vi "PH_Beamline_Chief.switch Exp Shutters.vi"(0 "i ref in":refnum<vi>, 1 "Status Subscriber Information before":T1, 5 "error in":errorcluster) -> (14 "i ref out":refnum<vi>, 19 "error out":errorcluster)   [LabVIEW 2014, in "PH_Beamline_Chief.lvlib"]
doc: "This VI sets the Switch GUI State GUI object."
uses:
  PH_Beamline_Chief.lvlib
  PH_Beamline/PH_Beamline.Status Subscriber Information.ctl
  PH_BL-Master/PH_BL-Master.Status Subscriber Information.ctl
  PH_BL-Master/PH_BL-Master.Attribute Set.ctl
  PH_Beamline/PH_Beamline.Switch Instances.ctl
  PH_Beamline/PH_Beamline.lvlib
  PH_Classes/PH_Switch/PH_Switch.lvlib
  PH_BL-Master/PH_BL-Master.lvlib
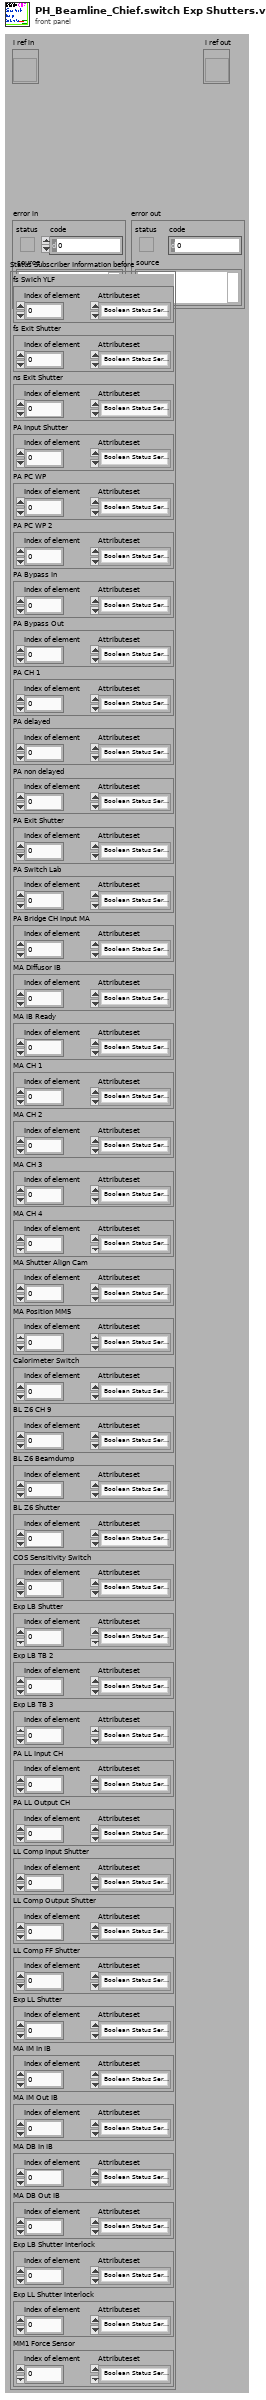
[diagram p1: front panel]
types:
  T1 = typedef "PH_Beamline.lvlib/PH_Beamline.Status Subscriber Information.ctl" = cluster{"fs Swich YLF":T2, "fs Exit Shutter":T2, "ns Exit Shutter":T2, "PA Input Shutter":T2, "PA PC WP":T2, "PA PC WP 2":T2, "PA Bypass In":T2, "PA Bypass Out":T2, "PA CH 1":T2, "PA delayed":T2, "PA non delayed":T2, "PA Exit Shutter":T2, "PA Switch Lab":T2, "PA Bridge CH Input MA":T2, "MA Diffusor IB":T2, "MA IB Ready":T2, "MA CH 1":T2, "MA CH 2":T2, "MA CH 3":T2, "MA CH 4":T2, "MA Shutter Align Cam":T2, "MA Position MM5":T2, "Calorimeter Switch":T2, "BL Z6 CH 9":T2, "BL Z6 Beamdump":T2, "BL Z6 Shutter":T2, "COS Sensitivity Switch":T2, "Exp LB Shutter":T2, "Exp LB TB 2":T2, "Exp LB TB 3":T2, "PA LL Input CH":T2, "PA LL Output CH":T2, "LL Comp Input Shutter":T2, "LL Comp Output Shutter":T2, "LL Comp FF Shutter":T2, "Exp LL Shutter":T2, "MA IM In IB":T2, "MA IM Out IB":T2, "MA DB In IB":T2, "MA DB Out IB":T2, "Exp LB Shutter Interlock":T2, "Exp LL Shutter Interlock":T2, "MM1 Force Sensor":T2}
  T2 = typedef "PH_BL-Master.lvlib/PH_BL-Master.Status Subscriber Information.ctl" = cluster{"Index of element":i32, "Attributeset":T3}
  T3 = typedef "PH_BL-Master.lvlib/PH_BL-Master.Attribute Set.ctl" = enum16{"Boolean Status Service Subscriber", "Picture Status Service Subscriber"}
  T4 = typedef "PH_Beamline.lvlib/PH_Beamline.Switch Instances.ctl" = string
  T5 = typedef "PH_Beamline.lvlib/PH_Beamline.i attribute.ctl" = cluster{"GUI Refs":cluster{"PA ok":refnum<vi>, "MA ok":refnum<vi>, "fs FE ok":refnum<vi>, "ns FE ok":refnum<vi>, "PA ED ok":refnum<vi>, "MAS ok":refnum<vi>, "Booster ok":refnum<vi>, "Mirrortower ok":refnum<vi>, "In.-Box ok":refnum<vi>, "Compressor ok":refnum<vi>, "Experiment LB ok":refnum<vi>, "Experiment LL ok":refnum<vi>, "PHELIX_Beckhoff_Watchdog":refnum<vi>, "Shutters closed":refnum<vi>, "uOPA ok":refnum<vi>, "Vacuum no shotcond Comp LB":refnum<vi>}, "Refs BL MA":refnum<vi>[], "Refs BL MA-IB":refnum<vi>[], "Refs BL fs":refnum<vi>[], "Refs BL PA ED":refnum<vi>[], "Refs BL MAS":refnum<vi>[], "Refs BL Boo":refnum<vi>[], "Refs BL ns":refnum<vi>[], "Refs BL Mirrortower":refnum<vi>[], "Refs BL Compressor":refnum<vi>[], "Refs BL Exp LB":refnum<vi>[], "Radiation Safety":cluster{"Exp Laserbay":cluster{"Ref Op Mode":refnum<vi>, "Ref Laserbay evacuated":refnum<vi>, "Tagname LB evacuated":string, "Shot Mode":T6, "Laserbay evacuated?":i32, "Tagname HV room locked":string, "HV room locked?":i32, "Ref HV room locked":refnum<vi>, "Tagname bridged?":string, "Ref Bridge":refnum<vi>, "I<1E18W/cm²":bool}, "Exp Laserlab":cluster{"Ref Op Mode":refnum<vi>, "Ref Laserlab evacuated":refnum<vi>, "Tagname LL evacuated":string, "Shot Mode":T6, "Laserlab evacuated?":i32, "Tagname bridged?":string, "Ref Bridge":refnum<vi>, "I<1E18W/cm²":bool}}, "Refs BL LL":refnum<vi>[], "PP Igni Heating GUI Refs":refnum<vi>[], "PP Igni Heating Tagnames ":string[], "Refs BL PA":cluster{"undelayed Line before Shutter":refnum<vi>[], "undelayed Line after Shutter":refnum<vi>[], "before Bypass":refnum<vi>[], "delayed Line before Shutter":refnum<vi>[], "delayed Line after Shutter":refnum<vi>[], "before Shutter Input":refnum<vi>[], "after Shutter Input":refnum<vi>[], "Bypass":refnum<vi>[], "before Shutter Exit":refnum<vi>[], "after Shutter Exit":refnum<vi>[], "to MA":refnum<vi>[], "to Lab":refnum<vi>[]}, "BL":cluster{"YLF_BL_Status":i32, "fs_BL_Status":i32, "fs_YLF_BL_Status":i32, "ns_BL_Status":i32, "PA_Input_BL_Status":i32, "PA_UnDelay_BL_Status":i32, "PA_Delay_BL_Status":i32, "PA_BL_Status":i32, "PA_Bypass_BL_Status":i32, "PA_Exit_BL_Status":i32, "PA_LL_BL_Status":i32, "LL_BL_Status":i32, "PA_MA_BL_Status":i32, "MA_Exit_BL_Status":i32, "MA_Z6_BL_Status":i32, "Z6_BL_Status":i32, "MA_LB_BL_Status":i32, "LB_TB2_BL_Status":i32, "PA_before_Bypass_BL_Status":i32, "LB_TB3_BL_Status":i32}, "State Subsystems":cluster{"PA":bool, "MA":bool, "ns FE":bool, "fs FE":bool, "PA ED":bool, "In.-Box":bool, "MAS":bool, "Booster":bool, "Mirrortower":bool, "Compressor":bool, "Experiment LB":bool, "Experiment LL":bool, "uOPA":bool}, "Status Subscriber Information":T1, "Refs BL uOPA":refnum<vi>[], "PA_Input_2_Beam_6PWpGUI not linked?":bool, "PA_Input_Delay_6PGUI not linked?":bool, "Settings":T7}
  T6 = typedef "PH_Beamline.lvlib/PH_Beamline.Operation Mode.ctl" = i32
  T7 = typedef "PH_Beamline_Chief.lvlib/PH_Beamline_Chief.Settings.ctl" = cluster{"PA Doublepass Mode":bool, "Compressor Vaccuum LB not relevant":bool, "Windowshutter TB2 not relevant":bool, "Windowshutter TB3 not relevant":bool}
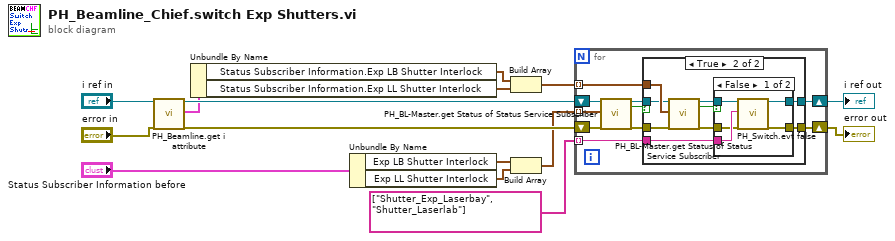
[diagram p0: block diagram]
diagram:
  n1 = call "PH_Beamline.get i attribute.vi"("i ref in"="i ref in", "error in (no error)"="error in") -> ("i ref out"=w12:refnum<vi>, "i attribute"=w10:T5, "error out"=w13:errorcluster)  [unwired: 15 in]
  n2 = Unbundle By Name(w10) -> ("Status Subscriber Information.Exp LB Shutter Interlock"=w9:T2, "Status Subscriber Information.Exp LL Shutter Interlock"=w1:T2)
  n3 = Unbundle By Name("Status Subscriber Information before") -> ("Exp LB Shutter Interlock"=w7:T2, "Exp LL Shutter Interlock"=w3:T2)
  n4 = Build Array(w9, w1) -> (w2:T2[])
  n5 = Build Array(w7, w3) -> (w4:T2[])
  n6 = for {
    tunnel: T4[] ["Shutter_Exp_Laserbay", "Shutter_Laserlab"] -> [w18] mode=indexing
    tunnel: w4 -> [w17] mode=indexing
    tunnel: w2 -> [w16] mode=indexing
    shift-right: [w24] -> w14
    shift-left: w13 -> [w23]
    shift-right: [w25] -> w15
    shift-left: w12 -> [w22]
    n7 = call "PH_BL-Master.get Status of Status Service Subscriber.vi"("i ref in"=w22, "Wanted Status Subscriber Information"=w17, "error in (no error)"=w23) -> ("i ref out"=w20:refnum<vi>, "off/false/out?"=w19:bool, "error out"=w21:errorcluster)  [unwired: 11 in, 3 out]
    n8 = case shown="True" w19 {
      tunnel: [w27 w36] -> w25
      tunnel: [w26 w35] -> w24
      tunnel: w16 -> [_ w34]
      tunnel: w21 -> [w26 w31]
      tunnel: w20 -> [w27 w30]
      tunnel: w18 -> [_ w28]
      frame False {
      }
      frame True {
        n9 = call "PH_BL-Master.get Status of Status Service Subscriber.vi"("i ref in"=w30, "Wanted Status Subscriber Information"=w34, "error in (no error)"=w31) -> ("i ref out"=w32:refnum<vi>, "off/false/out?"=w29:bool, "error out"=w33:errorcluster)  [unwired: 11 in, 3 out]
        n10 = case shown="False" w29 {
          tunnel: w33 -> [w38 w42]
          tunnel: [w37 w42] -> w35
          tunnel: [w39 w43] -> w36
          tunnel: w32 -> [w40 w43]
          tunnel: w28 -> [w41 _]
          frame False {
            n11 = call "PH_Switch.evt false.vi"("i ref in"=w40, "Instance"=w41, "error in (no error)"=w38) -> ("i ref out"=w39:refnum<vi>, "error out"=w37:errorcluster)  [unwired: 15 in]
          }
          frame True {
          }
        }
      }
    }
  }
  "error out" <- w14
  "i ref out" <- w15
